vi "Pixel 8 End Condition (SubVI).vi"(8 "Previous Fnd Location":u64, 10 "Contour Scan in":T1, 11 "Fnd?":bool) -> (2 "Contour Scan out":T1)   [LabVIEW 2015]
uses:
  Controls (FPGA)/Contour Scan.ctl
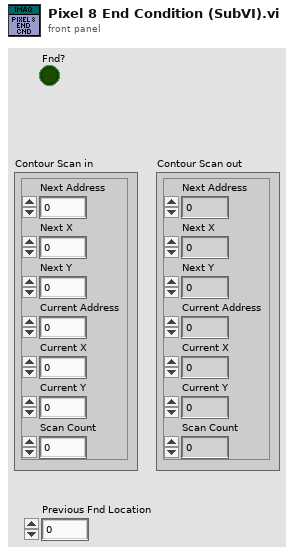
[diagram p1: front panel]
types:
  T1 = typedef "Contour Scan.ctl" = cluster{"Next Address":fxp<+,24,24>, "Next X":fxp<+,12,12>, "Next Y":fxp<+,12,12>, "Current Address":fxp<+,24,24>, "Current X":fxp<+,12,12>, "Current Y":fxp<+,12,12>, "Scan Count":u32}
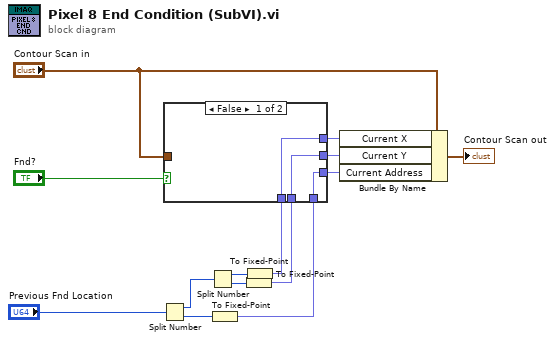
[diagram p0: block diagram]
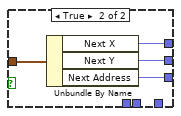
[diagram p2: hidden frame]
diagram:
  n1 = Split Number(x="Previous Fnd Location") -> (hi(x)=w7:u32, lo(x)=w4:u32)
  n2 = Split Number(x=w7) -> (hi(x)=w6:u16, lo(x)=w5:u16)
  n3 = To Fixed-Point(number=w4) -> (fixed-point=w1:fxp<+,24,24>)  [unwired: 1 in]
  n4 = To Fixed-Point(number=w5) -> (fixed-point=w2:fxp<+,12,12>)  [unwired: 1 in]
  n5 = To Fixed-Point(number=w6) -> (fixed-point=w3:fxp<+,12,12>)  [unwired: 1 in]
  n6 = case shown="False" "Fnd?" {
    tunnel: "Contour Scan in" -> [_ w21]
    tunnel: [w17 w20] -> w12
    tunnel: [w16 w19] -> w13
    tunnel: [w15 w18] -> w14
    tunnel: w3 -> [w17 _]
    tunnel: w2 -> [w16 _]
    tunnel: w1 -> [w15 _]
    frame False {
    }
    frame True {
      n7 = Unbundle By Name(w21) -> ("Next X"=w20:fxp<+,12,12>, "Next Y"=w19:fxp<+,12,12>, "Next Address"=w18:fxp<+,24,24>)
    }
  }
  n8 = Bundle By Name(cluster="Contour Scan in", "Current X"=w12, "Current Y"=w13, "Current Address"=w14) -> (→"Contour Scan out":T1)
